vi "IV Main.vi"() -> ()   [LabVIEW 2014]
panel:
  out "s":dbl[](array[numeric]) format="%.2f"
  out "Waveform Graph":dbl[](graph)
  out "status 2":i32 format="%.0x"
  in  "start":dbl step=1.0 format="%.2p"
  in  "speed":i32(slide)=2
  in  "number of points":i32=100 min=1 max=2500 step=1
  in  "source compliance":dbl min=-1100.0 max=1100.0 step=1.0 format="%.2p"
  in  "direction":i32(slide)
  in  "spacing":i32(slide)
  in  "ranging":i32(slide)
  in  "stop":dbl format="%.4f"
  in  "sense range":i32(slide)
  in  "size of reading":u32
  out "status":i32 format="%.0x"
  in  "resource name 2":string="GPIB0::24::INSTR"
  out "error out":errorcluster
  in  "resource name":string="ASRL4::INSTR"
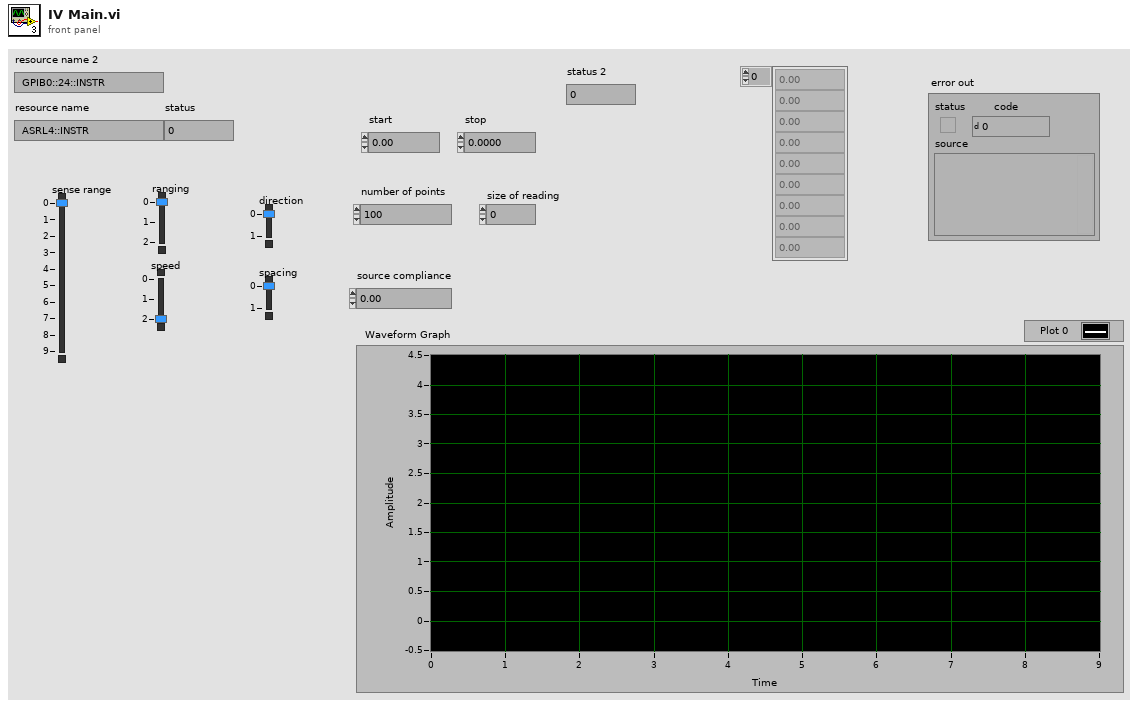
[diagram p1: front panel]
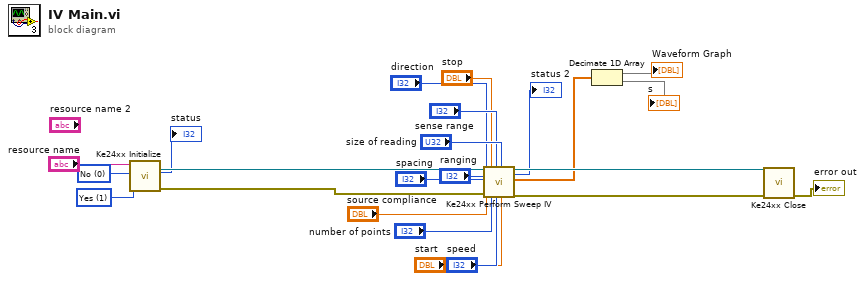
[diagram p0: block diagram]
diagram:
  w22 = u16 1 items=["Yes"=1, "No"=0] ("id query")
  w23 = u16 0 items=["Yes"=1, "No"=0] ("reset device")
  n1 = call <instrlib>:"Ke24xx Initialize.vi"("reset device"=w23, "id query"=w22, "resource name"="resource name") -> ("error out"=w16:errorcluster, "status"=→"status":i32, "instrument handle out"=w17:refnum<visa-resource-name>)  [unwired: 6 in]
  n2 = call <instrlib>:"Ke24xx Perform Sweep IV.vi"("instrument handle"=w17, "ranging"="ranging", "spacing"="spacing", "direction"="direction", "source compliance"="source compliance", "error in (no error)"=w16, "stop"="stop", "number of points"="number of points", "sense range"="sense range", "speed"="speed", "size of reading"="size of reading", "start"="start") -> ("instrument handle out"=w19:refnum<visa-resource-name>, "status"=→"status 2":i32, "s"=w3:dbl[], "error out"=w18:errorcluster)  [unwired: 4 in]
  n3 = Decimate 1D Array(w3) -> (→"Waveform Graph":dbl[], →"s":dbl[])
  n4 = call <instrlib>:"Ke24xx Close.vi"("error in (no error)"=w18, "instrument handle"=w19) -> ("error out"=→"error out":errorcluster)  [unwired: 8 in, 1 out]
